vi "Logical show tiered panel.vi"(8 "error in (no error)":errorcluster, 11 "Model Panel Logic in":refnum<class "Model Panel Logic.lvclass">) -> (0 "error out":errorcluster, 2 "Show tiered panel?":bool, 3 "Model Panel Logic out":refnum<class "Model Panel Logic.lvclass">)   [LabVIEW 2020, in "Form Model Interfaces.lvlib" / "Model Panel Logic.lvclass"]
uses:
  Model Panel Logic.lvclass
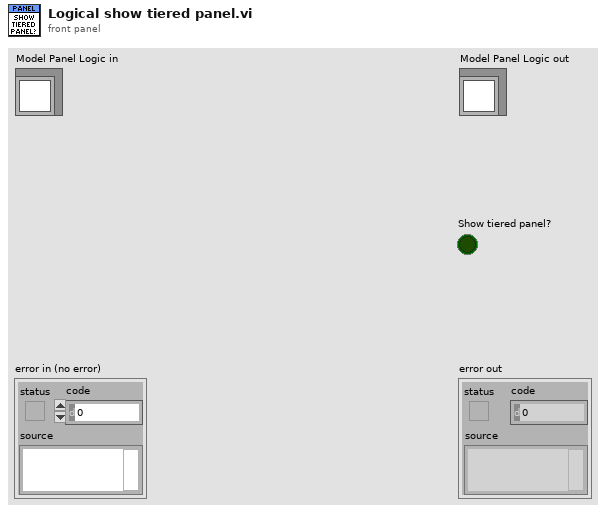
[diagram p1: front panel]
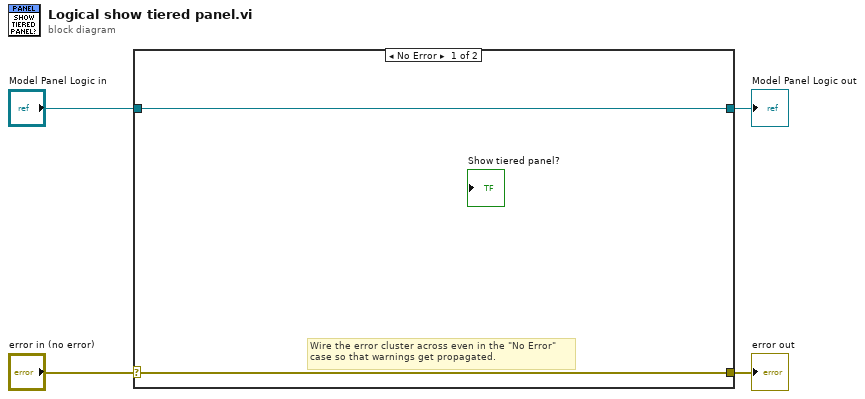
[diagram p0: block diagram]
diagram:
  n1 = case shown="No Error" "error in (no error)" {
    selector: "error in (no error)" -> [w5 w8]
    tunnel: [w5 w8] -> w3
    tunnel: [w6 w7] -> w1
    tunnel: "Model Panel Logic in" -> [w6 w7]
    frame No Error {
      # "Wire the error cluster across even in the \"No Error\"\ncase so that warnings get propagated."
    }
    frame Error {
    }
  }
  "error out" <- w3
  "Model Panel Logic out" <- w1
